vi "w0 via 2nd mom 1D.vi"(9 "Sum":ext, 10 "Input array":sgl[](array[numeric]), 11 "Centroid":sgl) -> (3 "w0 via 2nd mom":sgl)   [LabVIEW 2020]
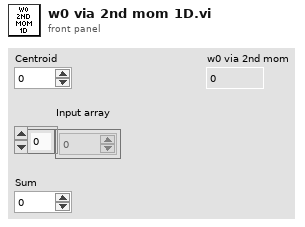
[diagram p1: front panel]
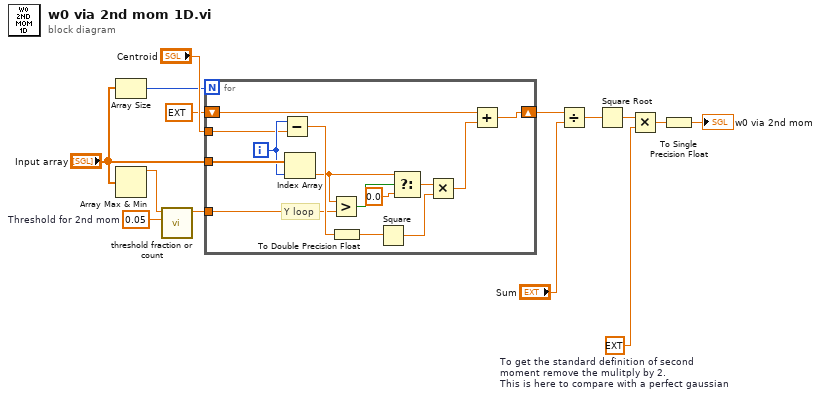
[diagram p0: block diagram]
diagram:
  w13 = 0.05  # Threshold for 2nd mom
  w6 = ext 2.0  # To get the standard definition of second moment remove the mulitply by 2. This is here to compare with a perfect gaussian
  n1 = Array Size(array="Input array") -> (size(s)=w2:i32)
  n2 = Array Max & Min(array="Input array") -> (max value=w12:sgl)  [unwired: 3 out]
  n3 = call "threshold fraction or count.vi"("Threshold in"=w13, "Maximal Value"=w12) -> ("Threshold out"=w14:dbl)  [unwired: 9 in]
  n4 = for {
    N: w2 -> [_]
    tunnel: "Input array" -> [w28]
    tunnel: "Centroid" -> [w26]
    shift-right: [w22] -> w7
    shift-left: ext 0.0 -> [w21]
    tunnel: w14 -> [w19]
    i -> [w27]
    # "Y loop"
    n5 = Subtract(x=w27, y=w26) -> (x-y=w25:sgl)
    n6 = Index Array(array=w28, index=w27) -> (element=w17:sgl)
    n7 = Greater?(x=w17, y=w19) -> (0:w18:bool)
    n8 = To Double Precision Float(number=w25) -> (double precision float=w20:dbl)
    n9 = Square(x=w20) -> (x^2=w24:dbl)
    n10 = Select(t=w17, s=w18, f=sgl 0.0) -> (s? t:f=w16:sgl)
    n11 = Multiply(x=w16, y=w24) -> (x*y=w23:dbl)
    n12 = Add(x=w21, y=w23) -> (x+y=w22:ext)
  }
  n13 = Divide(x=w7, y="Sum") -> (x/y=w5:ext)
  n14 = Square Root(x=w5) -> (sqrt(x)=w4:ext)
  n15 = Multiply(x=w4, y=w6) -> (x*y=w9:ext)
  n16 = To Single Precision Float(number=w9) -> (single precision float=→"w0 via 2nd mom":sgl)
